vi "Instrument.logToDatabaseMultiline.vi"(6 "timestamps":timestamp[](array[timestamp]), 8 "error in (no error)":errorcluster, 9 "Data":variant=variant(bool FALSE), 10 "Paths":string, 11 "Instrument":refnum<class "Instrument.lvclass">) -> (0 "error out":errorcluster, 3 "Instrument out":refnum<class "Instrument.lvclass">)   [LabVIEW 2019, in "Instrument.lvlib" / "Instrument.lvclass"]
doc: "Log data to database\n<b>Paths</b> is a path or list of paths\n<b>Data</b> object containing data to log, typically contained in a cluster if logging multiple items"
uses:
  Instrument.lvclass
  Typedefs/PrivateEvents--Instrument.LogDataMultiline.ctl
panel:
  # "For instructions on how to use the JKI State Machine Objects, examples and video tutorials, visit:\nhttp://jki.net/state-machine-objects/\n\nJKI State Machine Objects™\nhttp://jki.net/state-machine-objects/\nCopyright (C) 2005-2015, JKI <info@jki.net>\nALL RIGHTS RESERVED"
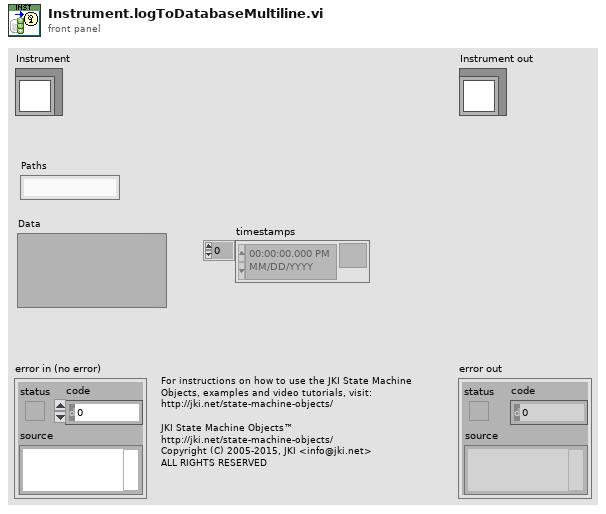
[diagram p1: front panel]
types:
  T1 = typedef "Instrument.lvlib/Instrument.lvclass/PrivateEvents--Instrument.LogDataMultiline.ctl" = cluster{"path":string, "data":variant, "timestamps":timestamp[]}
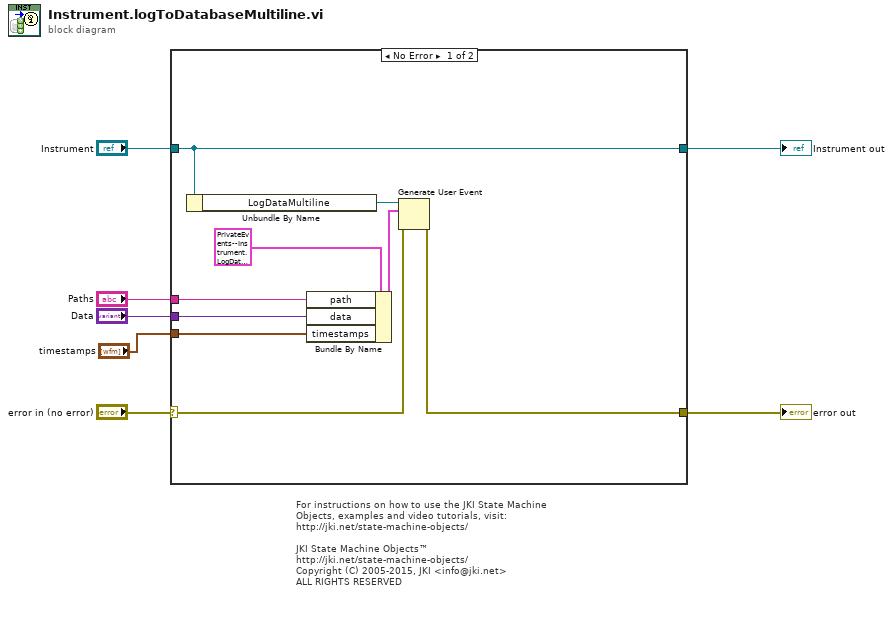
[diagram p0: block diagram]
diagram:
  # "For instructions on how to use the JKI State Machine Objects, examples and video tutorials, visit:\nhttp://jki.net/state-machine-objects/\n\nJKI State Machine Objects™\nhttp://jki.net/state-machine-objects/\nCopyright (C) 2005-2015, JKI <info@jki.net>\nALL RIGHTS RESERVED"
  n1 = case shown="No Error" "error in (no error)" {
    selector: "error in (no error)" -> [w16 w18]
    tunnel: [w14 w18] -> w6
    tunnel: [w13 w17] -> w7
    tunnel: "Instrument" -> [w13 w17]
    tunnel: "Paths" -> [w11 _]
    tunnel: "Data" -> [w10 _]
    tunnel: "timestamps" -> [w8 _]
    frame No Error {
      n2 = Unbundle By Name(w13) -> ("LogDataMultiline"=w15:refnum<user-event>)
      n3 = Bundle By Name(cluster=T1 {"path"="", "data"=variant, "timestamps"=[]} ("DataMultilineToLog"), "path"=w11, "data"=w10, "timestamps"=w8) -> (w12:T1)
      n4 = Generate User Event(user event=w15, event data cluster=w12, error in=w16) -> (error out=w14:errorcluster)  [unwired: 1 in, 1 out]
    }
    frame Error {
    }
  }
  "error out" <- w6
  "Instrument out" <- w7
